vi "Read Waveforms.vi"   [LabVIEW 2015, in "Agilent 2000 3000 X-Series.lvlib"]
doc: "Reads waveforms data."
uses:
  Agilent 2000 3000 X-Series.lvlib
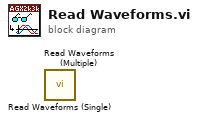
[diagram p0: block diagram]
diagram:
  n1 = call "Read Waveforms (Single).vi"() -> ()  [unwired: 9 in, 3 out]
  n2 = call "Read Waveforms (Multiple).vi"() -> ()  [unwired: 9 in, 3 out]
